vi "时间差（秒）.vi"(9 "Start Time":timestamp, 11 "End Time":timestamp) -> (3 "Seconds":dbl)   [LabVIEW 2012]
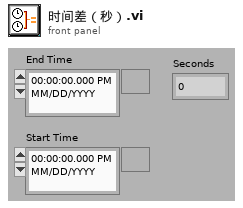
[diagram p1: front panel]
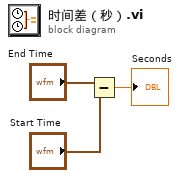
[diagram p0: block diagram]
diagram:
  n1 = Subtract(x="End Time", y="Start Time") -> (x-y=→"Seconds":dbl)
